vi "Get Tag.vi"(8 "error in (no error)":errorcluster, 9 "default value":variant, 10 "tag (case insensitive)":string, 11 "uData in":refnum<class "uData.lvclass">) -> (0 "error out":errorcluster, 1 "value":variant, 3 "uData out":refnum<class "uData.lvclass">, 4 "found?":bool)   [LabVIEW 2023, in "uData.lvlib" / "uData.lvclass"]
doc: "Read a tag."
uses:
  uData.lvclass
  uData.lvclass/uData.ctl
  Blank Key Reserved String.vi
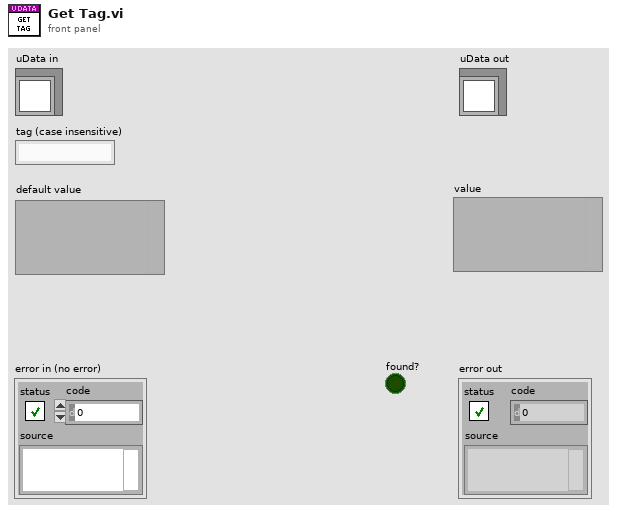
[diagram p1: front panel]
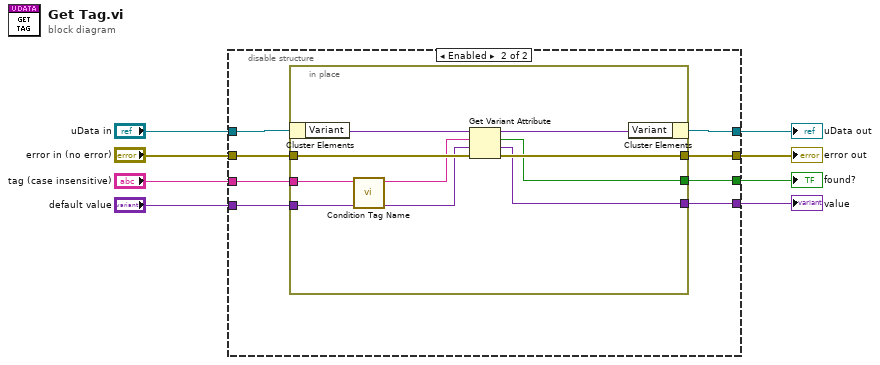
[diagram p0: block diagram]
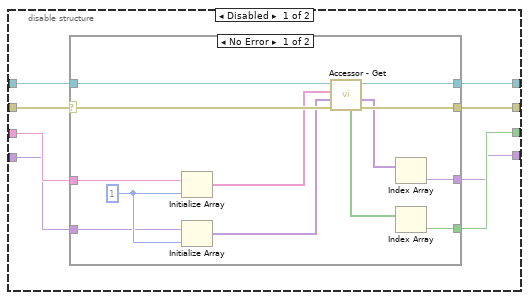
[diagram p2: hidden frame]
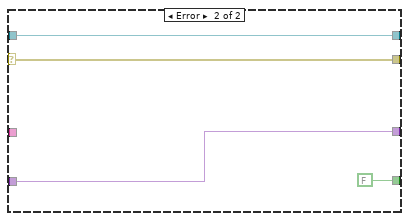
[diagram p3: hidden frame]
diagram:
  n1 = disable-structure shown="Enabled" {
    disable-tunnel: "uData in" -> [w16 w39]
    disable-tunnel: [w15 w34] -> w7
    disable-tunnel: [w14 w40] -> w6
    disable-tunnel: [w13 w35] -> w5
    disable-tunnel: "tag (case insensitive)" -> [w12 w38]
    disable-tunnel: "default value" -> [w11 w37]
    disable-tunnel: "error in (no error)" -> [w10 w41]
    disable-tunnel: [w9 w36] -> w1
    frame Disabled {
      n2 = case shown="No Error" w10 {
        selector: w10 -> [w28 w33]
        tunnel: w16 -> [w27 w32]
        tunnel: [w26 w32] -> w15
        tunnel: [w29 w33] -> w14
        tunnel: [w23 FALSE ("replaced")] -> w13
        tunnel: w12 -> [w20 _]
        tunnel: w11 -> [w18 w30]
        tunnel: [w22 w30] -> w9
        frame No Error {
          w24 = 1 ("dimension size")
          n3 = Initialize Array(w20, w24) -> (w19:string[])
          n4 = Initialize Array(w18, w24) -> (w17:variant[])
          n5 = call "Accessor - Get.vi"("error in (no error)"=w28, "default values"=w17, "keys"=w19, "uData in"=w27) -> ("error out"=w29:errorcluster, "values"=w21:variant[], "uData out"=w26:refnum<class "uData.lvclass">, "found?"=w25:bool[])  [unwired: 4 in]
          n6 = Index Array(array=w21) -> (element=w22:variant)  [unwired: 1 in]
          n7 = Index Array(array=w25) -> (element=w23:bool)  [unwired: 1 in]
        }
        frame Error {
        }
      }
    }
    frame Enabled {
      n8 = in-place {
        in-place-border: w41 -> [w50]
        in-place-border: [w49] -> w40
        in-place-border: w38 -> [w46]
        in-place-border: w37 -> [w45]
        in-place-border: [w44] -> w36
        in-place-border: [w43] -> w35
        n9 = in-place-cluster #1(w39) -> ("Variant"=w48:variant)
        n10 = call "Condition Tag Name.vi"("tag in"=w46) -> ("tag out"=w42:string)  [unwired: 10 in]
        n11 = Get Variant Attribute(Variant=w48, name=w42, default value (empty Variant)=w45, error in=w50) -> (duplicate Variant=w47:variant, found=w43:bool, value=w44:variant, error out=w49:errorcluster)
        n12 = in-place-cluster #1("Variant"=w47) -> (w34:refnum<class "uData.lvclass">)
      }
    }
  }
  "error out" <- w6
  "uData out" <- w7
  "found?" <- w5
  "value" <- w1
